vi "Button Handler.vi"(8 "error in (no error)":errorcluster, 9 "Buttons":bool[](array[boolean])) -> (0 "error out":errorcluster)   [LabVIEW 2016]
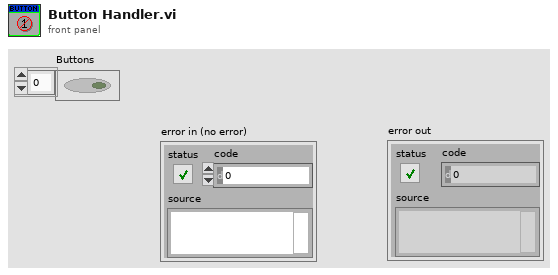
[diagram p1: front panel]
types:
  T1 = typedef "WPI_MotorControlDeviceRef.ctl" = cluster{"DeviceStatus":errorcluster, "Type":T2, "PWM":cluster{"PWM Channel":T3, "DeadBand":T4}, "CAN":cluster{"Device Number":u8, "SetOutput VI Ref":variant, "GetOutput VI Ref":variant, "Enable VI Ref":variant, "Disable VI Ref":variant, "Data":variant}, "Invert":bool}
  T2 = typedef "WPI_MotorControlType.ctl" = enum16{"PWM", "CAN"}
  T3 = typedef "FPGA_DIOPWMChannel.ctl" = enum8{"PWM 0", "PWM 1", "PWM 2", "PWM 3", "PWM 4", "PWM 5", "PWM 6", "PWM 7", "PWM 8", "PWM 9", "PWM MXP 0", "PWM MXP 1", "PWM MXP 2", "PWM MXP 3", "PWM MXP 4", "PWM MXP 5", "PWM MXP 6", "PWM MXP 7", "PWM MXP 8", "PWM MXP 9", "Invalid"}
  T4 = typedef "WPI_PWMDeadband.ctl" = cluster{"Name":string, "maxPositivePwm":i32, "minPositivePwm":i32, "centerPwm":i32, "maxNegativePwm":i32, "minNegativePwm":i32, "angularRange":u16}
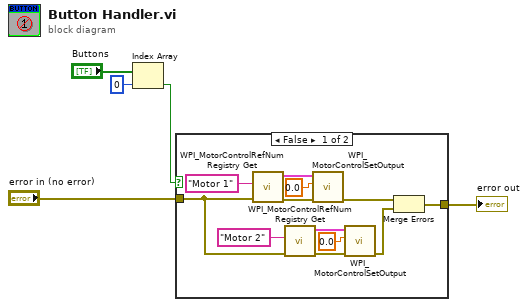
[diagram p0: block diagram]
diagram:
  n1 = Index Array(array="Buttons", index=0) -> (element=w2:bool)
  n2 = case shown="False" w2 {
    tunnel: "error in (no error)" -> [w11 w18]
    tunnel: [w6 w18] -> w1
    frame False {
      n3 = call <vilib>:"WPI_MotorControlRefNum Registry Get.vi"("error in (no error)"=w11, "refnum name"="Motor 1") -> ("error out"=w16:errorcluster, "MotorControlDevRef"=w15:T1)  [unwired: 8 in]
      n4 = call <vilib>:"WPI_MotorControlRefNum Registry Get.vi"("error in (no error)"=w11, "refnum name"="Motor 2") -> ("error out"=w13:errorcluster, "MotorControlDevRef"=w14:T1)  [unwired: 8 in]
      n5 = call <vilib>:"WPI_MotorControlSetOutput.vi"("error in (no error)"=w16, "Output"=0.0, "MotorControlDevRef"=w15) -> ("error out"=w8:errorcluster)  [unwired: 6 in, 2 out]
      n6 = call <vilib>:"WPI_MotorControlSetOutput.vi"("error in (no error)"=w13, "Output"=0.0, "MotorControlDevRef"=w14) -> ("error out"=w7:errorcluster)  [unwired: 6 in, 2 out]
      n7 = Merge Errors(w8, w7) -> (w6:errorcluster)
    }
    frame True {
    }
  }
  "error out" <- w1
